vi "Acquisition program_Scan and variance.vi"() -> ()   [LabVIEW 2019]
uses:
  <vilib>/Analysis/1siggen.llb/Ramp Pattern by Samples.vi
  <vilib>/Analysis/2dsp.llb/Real FFT.vi
  <vilib>/Utility/file.llb/Write Delimited Spreadsheet (DBL).vi
  <instrlib>/Stanford Research 830/Public/Data/Read (All Parameters).vi
  <instrlib>/Stanford Research 830/Stanford Research 830.lvlib
  <instrlib>/Zaber A Series/Zaber A Series.lvlib
  <vilib>/Analysis/NI_AALBase.lvlib
  <vilib>/Analysis/NI_AALPro.lvlib
panel:
  in  "?":T1(tab)=enum."Measurements"
  out "Y":dbl(graph)
  out "X":dbl(graph)
  in  "Delay (ps)":dbl=184.0
  out "to Position (mm)":dbl=27.572400000000002
  in  "Comments":string
  out "XY Graph":cluster{"Ramp Pattern":dbl[], dbl[]}[](graph)
  out "Scan #":i32
  in  "VISA Lock-In":refnum<visa-resource-name>="GPIB0::2::INSTR"
  in  "VISA Zaber":refnum<visa-resource-name>="COM6"
  in  "N points":i32=4096
  in  "Delay min (ps)":dbl min=0.0 max=339.0
  in  "Delay max (ps)":dbl=339.0 min=0.0 max=339.0
  in  "Number of Averages":i32=1
  in  "Wait (ms)":u32=100
  in  "?":bool
  out "Instrument ID":string="Stanford_Research_Systems,SR830,s/n81059,ver1.07"
  in  "Cancel":bool
  in  "?":bool
  out "Step Size (ps)":dbl=0.082763671875
  in  "measurements avg":i32=1
  in  "?":bool
  in  "Move Here":dbl=27.5724
  out "Current Position (mm)":dbl=27.5724
  in  "Position (mm)":dbl=50.8
  out "to Delay (ps)":dbl=339.0056723390056
  out "FFT X":cluster{dbl[], "FFT {X}":dbl[]}(graph)
  out "Power Spectra":cluster{dbl[], dbl[]}(graph)
  # "zero=27.36"
  # "ZERO=27.33"
  # "27.29"
  # "New zero!"
  # "27.565"
  # "27.6263"
  # "Conversions"
  # "27.5724\n11-02-2021"
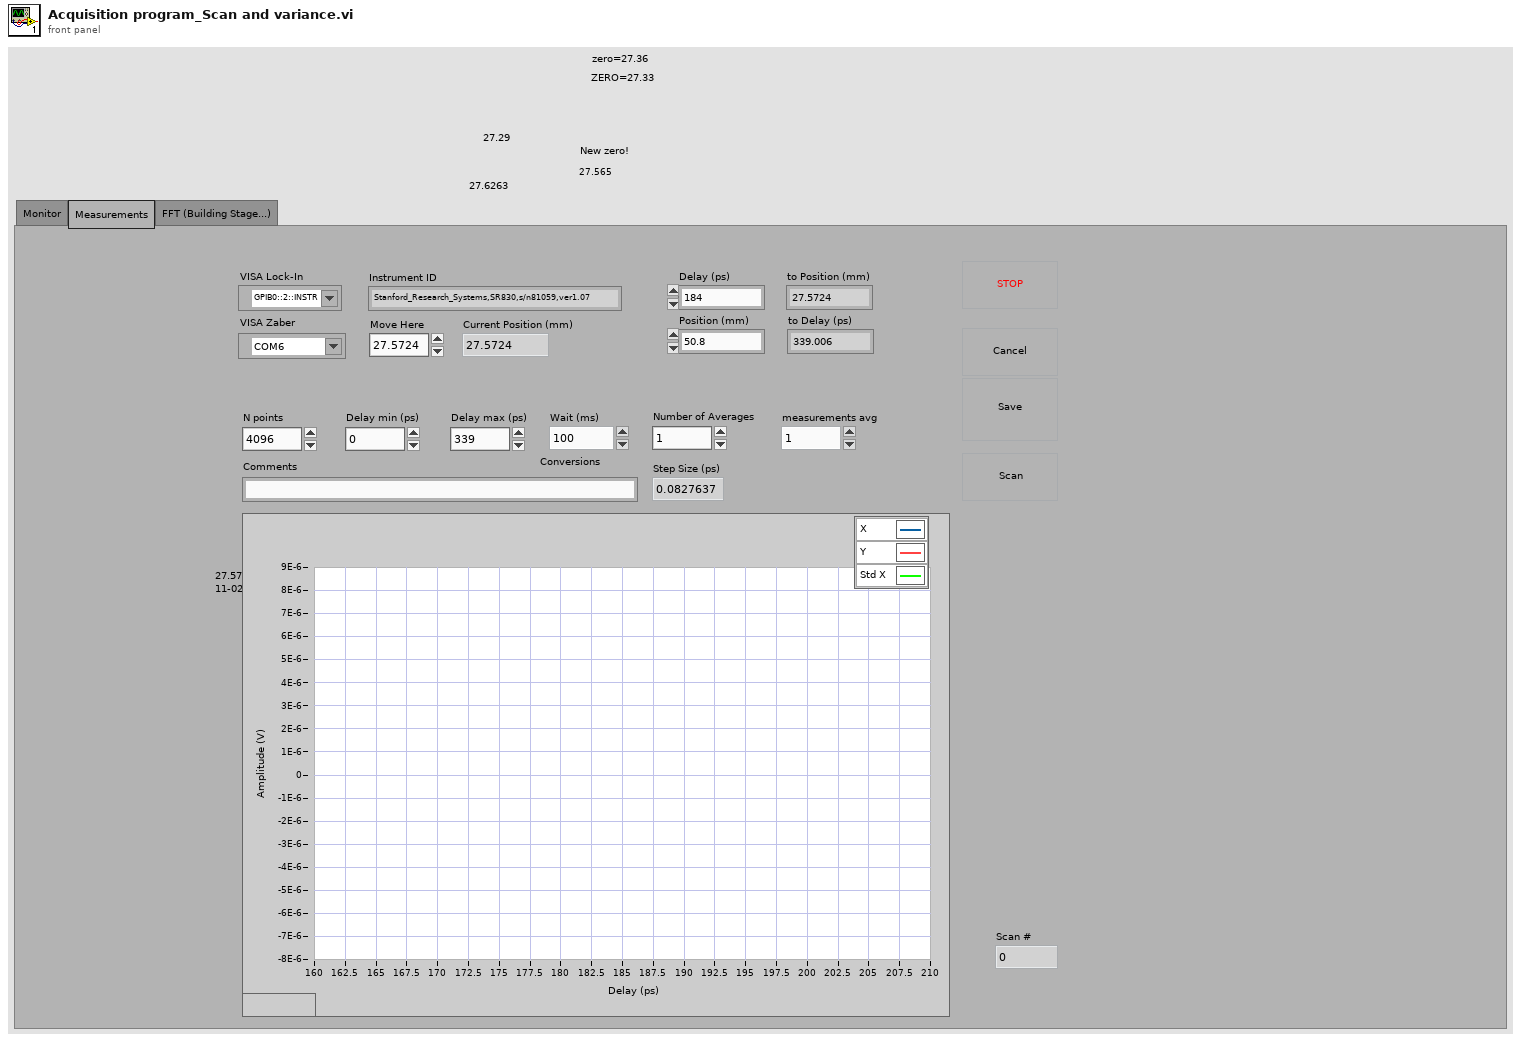
[diagram p1: front panel]
types:
  T1 = enum32{"Monitor", "Measurements", "FFT (Building Stage...)"}
  T2 = cluster{"X-Value":dbl, "Y-Value":dbl, "R-Value":dbl, "Theta-Value":dbl, "Aux In 1 Value":dbl, "Aux In 2 Value":dbl, "Aux In 3 Value":dbl, "Aux In 4 Value":dbl, "Reference Frequency":dbl, "Channel 1 Display":dbl, "Channel 2 Display":dbl}
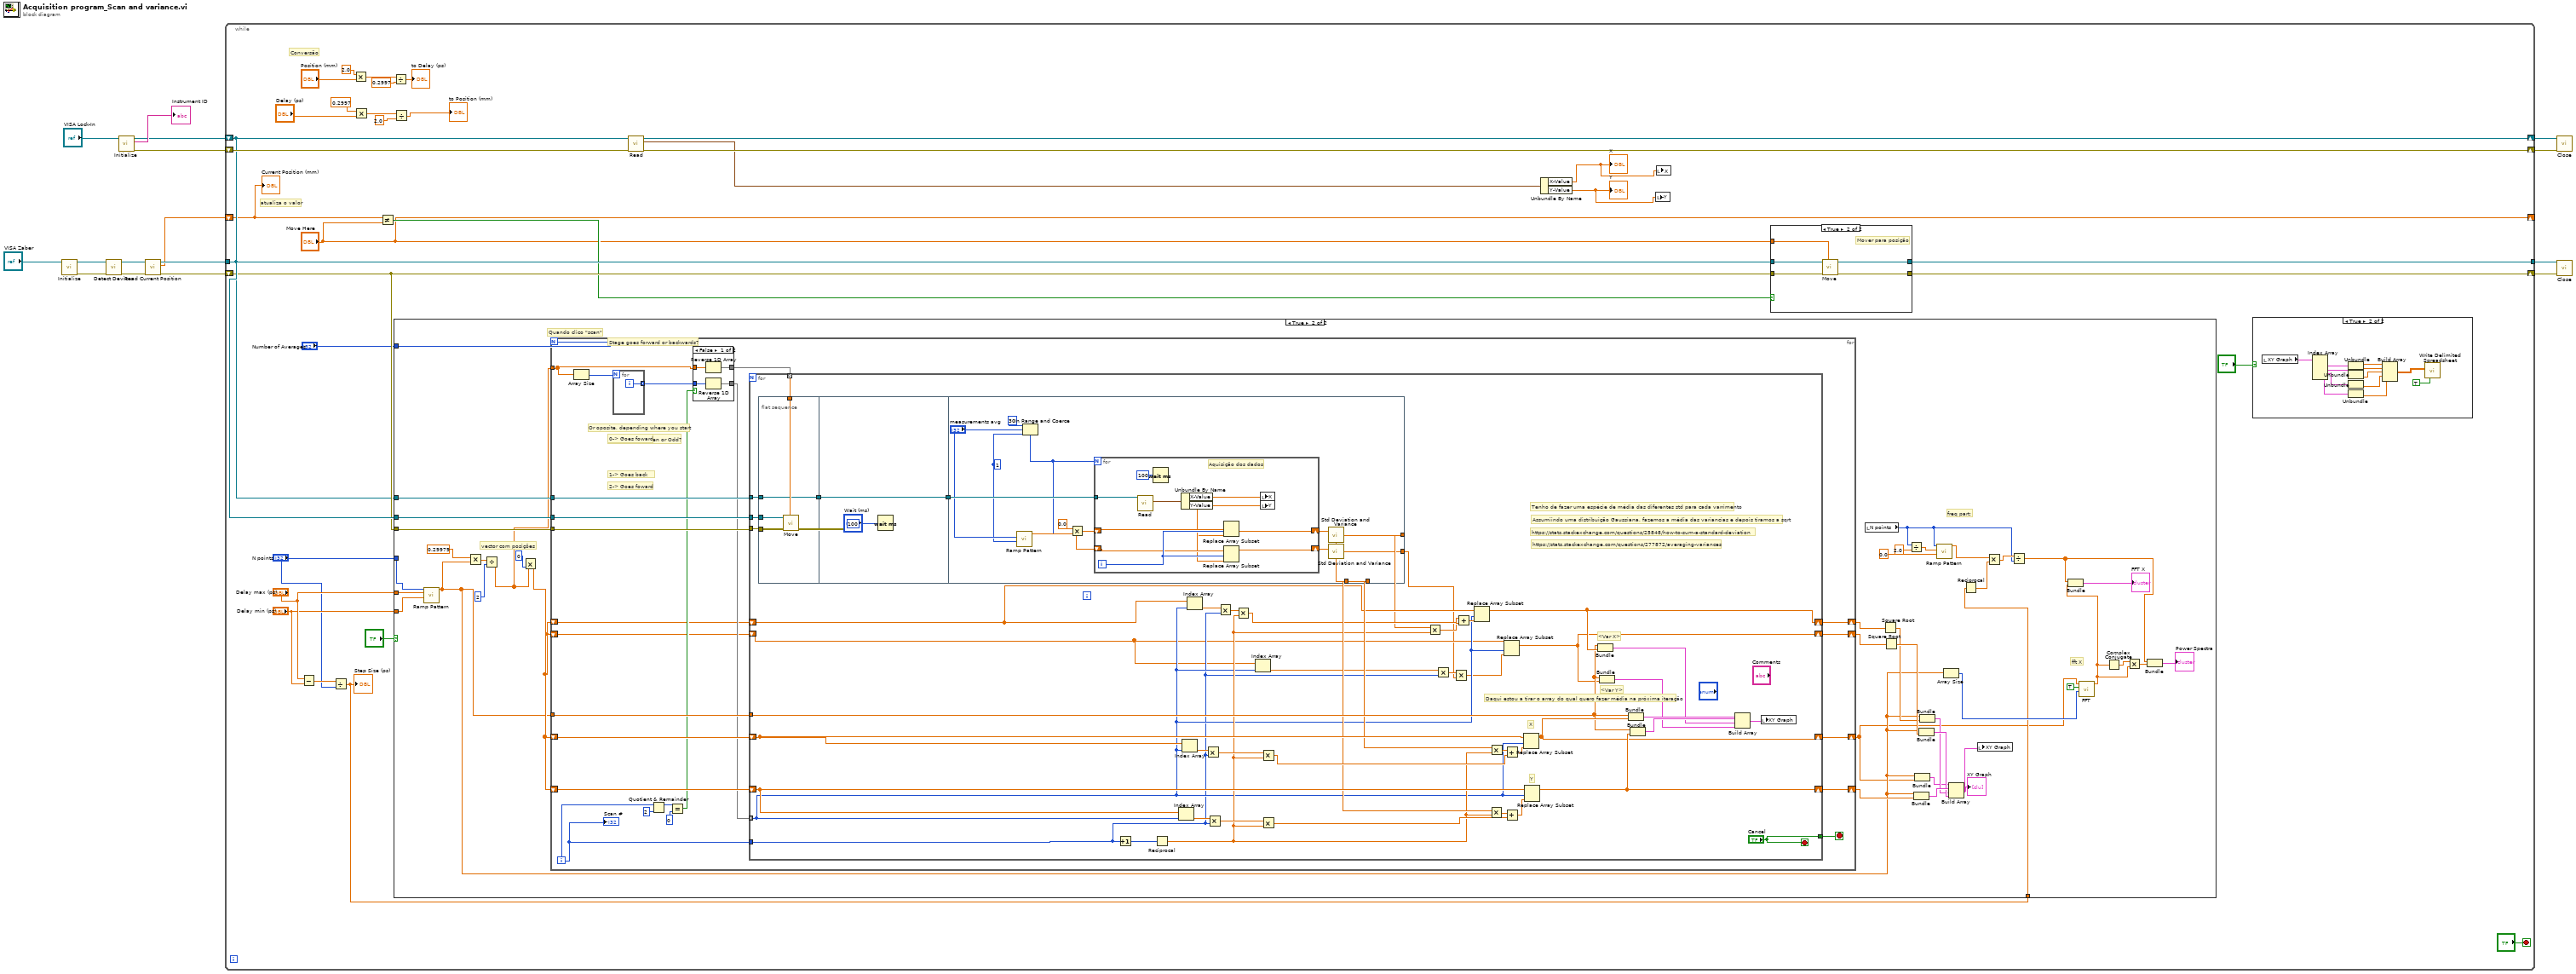
[diagram p0: block diagram]
diagram:
  n1 = call <instrlib>:"Initialize.vi"("VISA resource name"="VISA Zaber") -> ("error out"=w10:errorcluster, "VISA resource name out"=w11:refnum<visa-resource-name>)  [unwired: 9 in]
  n2 = call <instrlib>:"Detect Devices.vi"("error in (no error)"=w10, "VISA resource name"=w11) -> ("error out"=w8:errorcluster, "VISA resource name out"=w9:refnum<visa-resource-name>)  [unwired: 6 in, 2 out]
  n3 = call <instrlib>:"Initialize.vi"("VISA resource name"="VISA Lock-In") -> ("error out"=w2:errorcluster, "Instrument ID"=→"Instrument ID":string, "VISA resource name out"=w3:refnum<visa-resource-name>)  [unwired: 8 in]
  n4 = call <instrlib>:"Read Current Position.vi"("error in (no error)"=w8, "VISA resource name"=w9) -> ("error out"=w6:errorcluster, "Position"=w1:dbl, "VISA resource name out"=w7:refnum<visa-resource-name>)  [unwired: 7 in]
  n5 = while {
    shift-right: [w49] -> w14
    shift-left: w3 -> [w40]
    shift-right: [w47] -> w13
    shift-left: w2 -> [w48]
    tunnel: w7 -> [w42]
    tunnel: [w45] -> w5
    shift-right: [w44] -> w4
    shift-left: w6 -> [w41]
    shift-right: ["Move Here"] -> _
    shift-left: w1 -> [w23]
    stop <- "?" stop-if-true
    # "Conversão"
    # "atualiza o valor"
    n6 = Subtract(x="Delay max (ps)", y="Delay min (ps)") -> (x-y=w25:dbl)
    n7 = Divide(x=w25, y="N points") -> (x/y=w17:dbl)
    "Step Size (ps)" <- w17
    n8 = Multiply(x=2.0, y="Position (mm)") -> (x*y=w32:dbl)
    n9 = Multiply(x=0.2997, y="Delay (ps)") -> (x*y=w22:dbl)
    n10 = Not Equal?(x=w23, y="Move Here") -> (x != y?=w39:bool)
    n11 = Divide(x=w32, y=0.2997 ("x")) -> (x/y=→"to Delay (ps)":dbl)
    n12 = Divide(x=w22, y=2.0 ("x")) -> (x/y=→"to Position (mm)":dbl)
    n13 = case shown="True" "?" {
      tunnel: w42 -> [_ w102]
      tunnel: w41 -> [_ w101]
      tunnel: w40 -> [_ w100]
      tunnel: "Number of Averages" -> [_ w99]
      tunnel: "Delay min (ps)" -> [_ w97]
      tunnel: "Delay max (ps)" -> [_ w96]
      tunnel: "N points" -> [_ w95]
      tunnel: w17 -> [_ w76]
      frame False {
        # "Não clicar no scan"
      }
      frame True {
        # "fft X"
        # "freq part:"
        # "vector com posições"
        # "Quando clico \"scan\""
        n14 = call-poly <vilib>:"Ramp Pattern.vi"("start"=w97, "end"=w96, "samples"=w95) -> ("Ramp Pattern"=w80:dbl[])  [unwired: 7 in, 1 out]
        n15 = Multiply(x=0.29979, y=w80) -> (x*y=w91:dbl[])
        n16 = Divide(x=w91, y=2) -> (x/y=w89:dbl[])
        n17 = Multiply(x=w89, y=0) -> (x*y=w88:dbl[])
        n18 = for {
          N: w99 -> [_]
          tunnel: w102 -> [w115]
          tunnel: w101 -> [w125]
          tunnel: w100 -> [w124]
          tunnel: w80 -> [w121]
          tunnel: w89 -> [w113]
          shift-right: [w109] -> w68
          shift-left: w88 -> [w123]
          shift-right: [w108] -> w93
          shift-left: w88 -> [w122]
          shift-right: [w104] -> w87
          shift-left: w88 -> [w106]
          shift-right: [w103] -> w86
          shift-left: w88 -> [w105]
          i -> [w107]
          stop <- w110 stop-if-true
          # "Or oposite, depending where you start"
          # "2-> Goes foward"
          # "1-> Goes back"
          # "0-> Goes foward"
          # "Stage goes forward or backwards?"
          # "Scan Number Even or Odd?"
          n19 = Array Size(array=w113) -> (size(s)=w117:i32)
          n20 = for {
            N: w117 -> [_]
            tunnel: [w126] -> w116 mode=indexing
            i -> [w126]
          }
          n21 = Quotient & Remainder(x=w107, y=2) -> (x-y*floor(x/y)=w118:i32)  [unwired: 1 out]
          n22 = Equal?(x=w118, y=0) -> (x = y?=w114:bool)
          n23 = case shown="False" w114 {
            tunnel: w116 -> [w130 w132]
            tunnel: [w129 w132] -> w111
            tunnel: w113 -> [w128 w131]
            tunnel: [w127 w131] -> w112
            frame False {
              n24 = Reverse 1D Array(array=w128) -> (reversed array=w127:dbl[])
              n25 = Reverse 1D Array(array=w130) -> (reversed array=w129:i32[])
            }
            frame True {
            }
          }
          n26 = for {
            tunnel: w115 -> [w179]
            tunnel: w125 -> [w178]
            tunnel: w124 -> [w157]
            shift-right: [w161] -> w109
            shift-left: w123 -> [w167]
            shift-right: [w162] -> w108
            shift-left: w122 -> [w168]
            tunnel: w121 -> [w153]
            tunnel: w112 -> [w177] mode=indexing
            tunnel: w107 -> [w136]
            tunnel: w111 -> [w137] mode=indexing
            tunnel: ["Cancel"] -> w110
            shift-right: [w154] -> w104
            shift-left: w106 -> [w147]
            shift-right: [w152] -> w103
            shift-left: w105 -> [w135]
            stop <- "Cancel" stop-if-true
            # "https://stats.stackexchange.com/questions/277872/averaging-variances"
            # "https://stats.stackexchange.com/questions/25848/how-to-sum-a-standard-deviation"
            # "Assumiindo uma distribuição Gaussiana, fazemos a média das variancias e depois tiramos a sqrt"
            # "Tenho de fazer uma espécie de média das diferentes std para cada varrimento"
            # "<Var Y>"
            # "<Var X>"
            # "Y"
            # "X"
            # "Daqui estou a tirar o array do qual quero fazer média na próxima iteração"
            n27 = flat-sequence {
              tunnel: w179 -> [w183]
              tunnel: w178 -> [w182]
              tunnel: w177 -> [w181]
              tunnel: w157 -> [w180]
              tunnel: [w180] -> w156
              tunnel: w156 -> [w184]
              tunnel: [w184] -> w155
              tunnel: [w190] -> w149
              tunnel: [w189] -> w148
              tunnel: w155 -> [w199]
              tunnel: [w187] -> w141
              tunnel: [w186] -> w134
              frame #0 {
                n28 = call <instrlib>:"Move.vi"("Move Distance (0)"=w181, "error in (no error)"=w182, "VISA resource name"=w183) -> ()  [unwired: 7 in, 2 out]
              }
              frame #1 {
                n29 = Wait (ms)(milliseconds to wait=u32 100) -> ()  [unwired: 1 out]
              }
              frame #2 {
                w194 = 1
                n30 = In Range and Coerce(upper limit=30, x="measurements avg", lower limit=w194) -> (coerced(x)=w188:i32)  [unwired: 1 out]
                n31 = call-poly <vilib>:"Ramp Pattern.vi"("start"=w194, "end"="measurements avg", "samples"=w188) -> ("Ramp Pattern"=w196:dbl[])  [unwired: 7 in, 1 out]
                n32 = Multiply(x=0.0, y=w196) -> (x*y=w193:dbl[])
                n33 = for {
                  N: w188 -> [_]
                  tunnel: w199 -> [w208]
                  shift-right: [w206] -> w191
                  shift-left: w193 -> [w203]
                  shift-right: [w205] -> w192
                  shift-left: w193 -> [w204]
                  i -> [w207]
                  # "Aquisição dos dados"
                  n34 = call-poly <instrlib>:"Read.vi"("VISA resource name"=w208) -> ("Parameter Values"=w209:T2)  [unwired: 8 in, 2 out]
                  n35 = Wait (ms)(milliseconds to wait=u32 100) -> ()  [unwired: 1 out]
                  n36 = Unbundle By Name(w209) -> ("X-Value"=w200:dbl, "Y-Value"=w201:dbl)
                  n37 = Replace Array Subset(array=w204, new element=w201, index=w207) -> (w205:dbl[])
                  n38 = Replace Array Subset(array=w203, new element=w200, index=w207) -> (w206:dbl[])
                  n39 = local write "X"(w200) -> ()
                  n40 = local write "Y"(w201) -> ()
                }
                n41 = call <vilib>:"Std Deviation and Variance.vi"("X"=w191) -> ("mean"=w190:dbl, "variance"=w187:dbl)  [unwired: 1 in, 1 out]
                n42 = call <vilib>:"Std Deviation and Variance.vi"("X"=w192) -> ("mean"=w189:dbl, "variance"=w186:dbl)  [unwired: 1 in, 1 out]
              }
            }
            n43 = Increment(x=w136) -> (x+1=w175:i32)
            n44 = Reciprocal(x=w175) -> (1/x=w142:dbl)
            n45 = Index Array(array=w168, index=w137) -> (element=w174:dbl)
            n46 = Index Array(array=w167, index=w137) -> (element=w172:dbl)
            n47 = Index Array(array=w147, index=w137) -> (element=w146:dbl)
            n48 = Multiply(x=w172, y=w136) -> (x*y=w171:dbl)
            n49 = Multiply(x=w174, y=w136) -> (x*y=w173:dbl)
            n50 = Multiply(x=w146, y=w136) -> (x*y=w145:dbl)
            n51 = Multiply(x=w145, y=w142) -> (x*y=w144:dbl)
            n52 = Index Array(array=w135, index=w137) -> (element=w139:dbl)
            n53 = Multiply(x=w171, y=w142) -> (x*y=w163:dbl)
            n54 = Multiply(x=w173, y=w142) -> (x*y=w164:dbl)
            n55 = Multiply(x=w141, y=w142) -> (x*y=w143:dbl)
            n56 = Multiply(x=w139, y=w136) -> (x*y=w138:dbl)
            n57 = Multiply(x=w138, y=w134) -> (x*y=w133:dbl)
            n58 = Add(x=w143, y=w144) -> (x+y=w140:dbl)
            n59 = Replace Array Subset(array=w147, new element=w140, index=w137) -> (w154:dbl[])
            n60 = Multiply(x=w148, y=w142) -> (x*y=w170:dbl)
            n61 = Multiply(x=w149, y=w142) -> (x*y=w165:dbl)
            n62 = Replace Array Subset(array=w135, new element=w133, index=w137) -> (w152:dbl[])
            n63 = Add(x=w165, y=w163) -> (x+y=w166:dbl)
            n64 = Add(x=w170, y=w164) -> (x+y=w169:dbl)
            n65 = Replace Array Subset(array=w167, new element=w166, index=w137) -> (w161:dbl[])
            n66 = Replace Array Subset(array=w168, new element=w169, index=w137) -> (w162:dbl[])
            n67 = Bundle("Ramp Pattern"=w153, w154) -> (w151:cluster{"Ramp Pattern":dbl[], dbl[]})  [unwired: 1 in]
            n68 = Bundle("Ramp Pattern"=w153, w152) -> (w150:cluster{"Ramp Pattern":dbl[], dbl[]})  [unwired: 1 in]
            n69 = Bundle("Ramp Pattern"=w153, w161) -> (w160:cluster{"Ramp Pattern":dbl[], dbl[]})  [unwired: 1 in]
            n70 = Bundle("Ramp Pattern"=w153, w162) -> (w159:cluster{"Ramp Pattern":dbl[], dbl[]})  [unwired: 1 in]
            n71 = Build Array(w160, w159, w151, w150) -> (w158:cluster{"Ramp Pattern":dbl[], dbl[]}[])
            n72 = local write "XY Graph"(w158) -> ()
          }
          "Scan #" <- w107
        }
        n73 = local read "N points"() -> (w69:i32)
        n74 = Square Root(x=w87) -> (sqrt(x)=w84:dbl[])
        n75 = Square Root(x=w86) -> (sqrt(x)=w85:dbl[])
        n76 = Divide(x=w69, y=2.0) -> (x/y=w73:dbl)
        n77 = Bundle("Ramp Pattern"=w80, w93) -> (w94:cluster{"Ramp Pattern":dbl[], dbl[]})  [unwired: 1 in]
        n78 = Bundle("Ramp Pattern"=w80, w68) -> (w77:cluster{"Ramp Pattern":dbl[], dbl[]})  [unwired: 1 in]
        n79 = Bundle("Ramp Pattern"=w80, w85) -> (w83:cluster{"Ramp Pattern":dbl[], dbl[]})  [unwired: 1 in]
        n80 = Bundle("Ramp Pattern"=w80, w84) -> (w78:cluster{"Ramp Pattern":dbl[], dbl[]})  [unwired: 1 in]
        n81 = call-poly <vilib>:"Ramp Pattern.vi"("start"=0.0, "end"=w73, "samples"=w69) -> ("Ramp Pattern"=w72:dbl[])  [unwired: 7 in, 1 out]
        n82 = Array Size(array=w80) -> (size(s)=w79:i32)
        n83 = Build Array(w77, w94, w78, w83) -> (w82:cluster{"Ramp Pattern":dbl[], dbl[]}[])
        "XY Graph" <- w82
        n84 = Reciprocal(x=w76) -> (1/x=w71:dbl)
        n85 = local write "XY Graph"(w82) -> ()
        n86 = Multiply(x=w72, y=w71) -> (x*y=w70:dbl[])
        n87 = Divide(x=w70, y=w69) -> (x/y=w63:dbl[])
        n88 = call-poly <vilib>:"FFT.vi"("FFT size"=w79, "shift?"=TRUE, "X"=w68) -> ("FFT {X}"=w65:cdb[])  [unwired: 7 in, 1 out]
        n89 = Bundle(w63, "FFT {X}"=w65) -> (→"FFT X":cluster{dbl[], "FFT {X}":cdb[]})  [unwired: 1 in]
        n90 = Complex Conjugate(1:w65) -> (0:w66:cdb[])
        n91 = Multiply(x=w66, y=w65) -> (x*y=w64:cdb[])
        n92 = Bundle(w63, w64) -> (→"Power Spectra":cluster{dbl[], cdb[]})  [unwired: 1 in]
      }
    }
    n93 = call-poly <instrlib>:"Read.vi"("error in (no error)"=w48, "VISA resource name"=w40) -> ("error out"=w47:errorcluster, "Parameter Values"=w37:T2, "VISA resource name out"=w49:refnum<visa-resource-name>)  [unwired: 7 in]
    n94 = Unbundle By Name(w37) -> ("X-Value"=w29:dbl, "Y-Value"=w28:dbl)
    "X" <- w29
    "Y" <- w28
    n95 = local write "Y"(w28) -> ()
    n96 = local write "X"(w29) -> ()
    n97 = case shown="True" w39 {
      tunnel: w42 -> [w211 w216]
      tunnel: w41 -> [w210 w215]
      tunnel: [w211 w214] -> w45
      tunnel: [w210 w213] -> w44
      tunnel: "Move Here" -> [_ w212]
      frame False {
      }
      frame True {
        # "Mover para posição"
        n98 = call <instrlib>:"Move.vi"("Move Distance (0)"=w212, "error in (no error)"=w215, "VISA resource name"=w216) -> ("error out"=w213:errorcluster, "VISA resource name out"=w214:refnum<visa-resource-name>)  [unwired: 7 in]
      }
    }
    n99 = case shown="True" "?" {
      frame False {
      }
      frame True {
        n100 = local read "XY Graph"() -> (w61:cluster{"Ramp Pattern":dbl[], dbl[]}[])
        n101 = Index Array(array=w61) -> (element #1=w60:cluster{"Ramp Pattern":dbl[], dbl[]}, element #2=w59:cluster{"Ramp Pattern":dbl[], dbl[]}, element #3=w53:cluster{"Ramp Pattern":dbl[], dbl[]}, element #4=w52:cluster{"Ramp Pattern":dbl[], dbl[]})  [unwired: 4 in]
        n102 = Unbundle(w60) -> ("Ramp Pattern"=w58:dbl[], w57:dbl[])
        n103 = Unbundle(w59) -> (w56:dbl[])  [unwired: 1 out]
        n104 = Unbundle(w53) -> (w51:dbl[])  [unwired: 1 out]
        n105 = Unbundle(w52) -> (w50:dbl[])  [unwired: 1 out]
        n106 = Build Array(w58, w57, w56, w51, w50) -> (w55:dbl[][])
        n107 = call-poly <vilib>:"Write Delimited Spreadsheet.vi"("2D data"=w55, "transpose? (no:F)"=TRUE) -> ()  [unwired: 12 in, 2 out]
      }
    }
    "Current Position (mm)" <- w23
  }
  n108 = call <instrlib>:"Close.vi"("error in (no error)"=w13, "VISA resource name"=w14) -> ()  [unwired: 9 in, 1 out]
  n109 = call <instrlib>:"Close.vi"("error in (no error)"=w4, "VISA resource name"=w5) -> ()  [unwired: 9 in, 1 out]
